vi "Tusk.MessageTerminal.vi"(8 "error in (no error)":errorcluster, 11 "Tusk in":refnum<class "Tusk.lvclass">) -> (3 "Tusk out":refnum<class "Tusk.lvclass">, 4 "Stop?":bool)   [LabVIEW 2018, in "Application.lvlib" / "Tusk.lvclass"]
uses:
  Tusk.lvclass
  Tusk.lvclass/Tusk.ctl
  Message Class/Message.lvclass/Message.ctl
  Message Class/Message.lvclass
  Dictionary Class/Dictionary.lvclass/Dictionary.ctl
  Message Class/VIs/Wrap Message.vi
  Tusk.GetName (Local).vi
  Tusk.MessageAllSenderCore.vi
  Keywords Class/VIs/{All}.vi
  Tusk.GetDictionary.vi
  Tusk.MessageAllSenderCore.vi/1679c56e-e765-44f0-aff8-f47c4dbf3d60.vi
  Tusk.MessageSenderCore.vi
  Dictionary Class/VIs/Get Data DVR.vi
  Exceptions Class/VIs/Invalid Type.vi
  <vilib>/Utility/SystemLogging/Write to System Log.vi
  <vilib>/Utility/error.llb/Trim Whitespace.vi
  Keywords Class/Keywords.lvclass
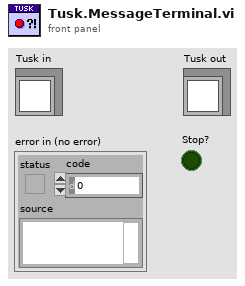
[diagram p1: front panel]
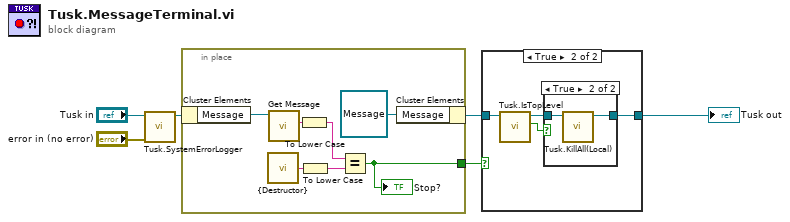
[diagram p0: block diagram]
diagram:
  n1 = call "Tusk.SystemErrorLogger.vi"("error in (no error)"="error in (no error)", "Tusk in"="Tusk in") -> ("Tusk out"=w4:refnum<class "Tusk.lvclass">)  [unwired: 8 in, 1 out]
  n2 = in-place {
    in-place-border: [w7] -> w2
    n3 = in-place-cluster #1(w4) -> ("Message"=w13:refnum<class "Message.lvclass">)
    n4 = call "{Destructor}.vi"() -> ("Word"=w10:string)  [unwired: 6 in]
    n5 = call "Get Message.vi"("Message in"=w13) -> ("Message"=w11:string)  [unwired: 8 in, 2 out]
    n6 = To Lower Case(string=w11) -> (all lower case string=w9:string)
    n7 = To Lower Case(string=w10) -> (all lower case string=w8:string)
    n8 = Equal?(x=w9, y=w8) -> (x = y?=w7:bool)
    "Stop?" <- w7
    n9 = in-place-cluster #1("Message"=refnum<class "Message.lvclass"> refnum) -> (w3:refnum<class "Tusk.lvclass">)
  }
  n10 = case shown="True" w2 {
    tunnel: w3 -> [w14 w16]
    tunnel: [w14 w15] -> w1
    frame False {
    }
    frame True {
      n11 = call "Tusk.IsTopLevel.vi"("Tusk in"=w16) -> ("Is Top Level?"=w18:bool, "Tusk out"=w17:refnum<class "Tusk.lvclass">)  [unwired: 8 in, 1 out]
      n12 = case shown="True" w18 {
        tunnel: w17 -> [w19 w21]
        tunnel: [w19 w20] -> w15
        frame False {
        }
        frame True {
          n13 = call "Tusk.KillAll(Local).vi"("Tusk in"=w21) -> ("Tusk out"=w20:refnum<class "Tusk.lvclass">)  [unwired: 9 in, 1 out]
        }
      }
    }
  }
  "Tusk out" <- w1
